vi "Save Data.vi"(8 "error in (no error)":errorcluster, 10 "signal out":waveform(dbl), 11 "Loggin in":refnum<class "Loggin.lvclass">) -> (0 "error out":errorcluster, 3 "Loggin out":refnum<class "Loggin.lvclass">)   [LabVIEW 2020, in "Loggin.lvlib" / "Loggin.lvclass"]
uses:
  Loggin.lvclass
  Loggin.lvclass/Loggin.ctl
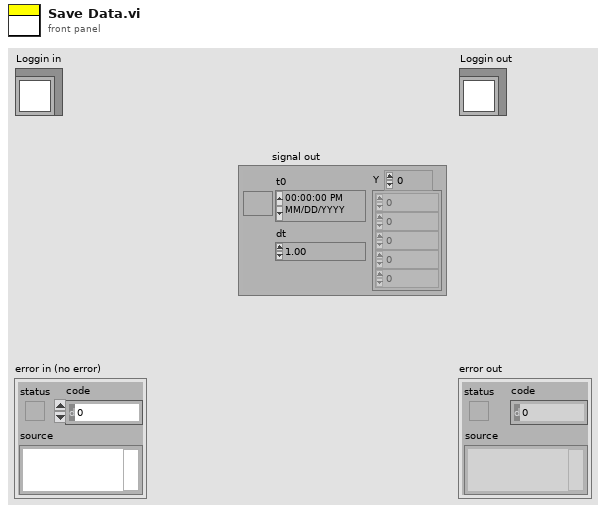
[diagram p1: front panel]
types:
  T1 = enum16{"open", "replace", "create", "open or create", "replace or create", "replace or create with confirmation"}
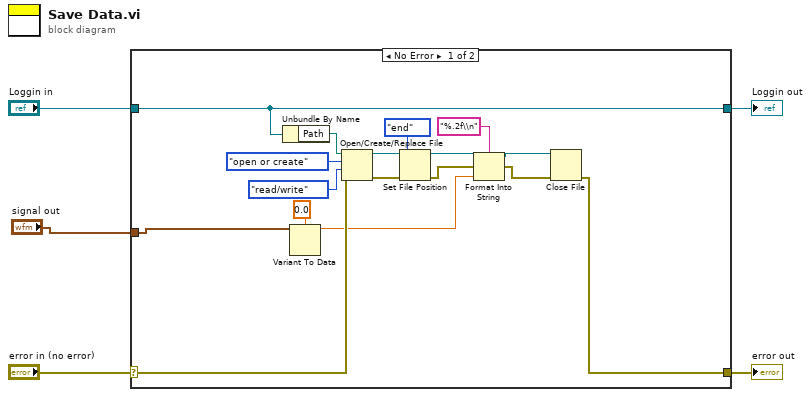
[diagram p0: block diagram]
diagram:
  n1 = case shown="No Error" "error in (no error)" {
    selector: "error in (no error)" -> [w10 w24]
    tunnel: [w9 w24] -> w4
    tunnel: [w11 w23] -> w2
    tunnel: "Loggin in" -> [w11 w23]
    tunnel: "signal out" -> [w8 _]
    frame No Error {
      n2 = Unbundle By Name(w11) -> ("Path"=w22:path)
      n3 = Variant To Data(type=0.0, Variant=w8) -> (data=w6:dbl)  [unwired: 1 in, 1 out]
      n4 = Open/Create/Replace File(file path (use dialog)=w22, error in=w10, operation (0:open)=T1."open or create", access (0:read/write)=enum16{"read/write", "read-only", "write-only"}."read/write") -> (refnum out=w16:refnum<file>, error out=w17:errorcluster)  [unwired: 2 in, 1 out]
      n5 = Set File Position(refnum=w16, from (0:start)=enum16{"start", "end", "current"}."end", error in=w17) -> (refnum out=w15:refnum<file>, error out=w14:errorcluster)  [unwired: 1 in]
      n6 = Format Into String(format string="%.2f\\n", initial string=w15, error in=w14, w6) -> (resulting string=w19:refnum<file>, error out=w18:errorcluster)
      n7 = Close File(refnum=w19, error in=w18) -> (error out=w9:errorcluster)  [unwired: 1 out]
    }
    frame Error {
    }
  }
  "error out" <- w4
  "Loggin out" <- w2
